vi "Write (Timestamp).vi"(9 "error in (no error)":errorcluster, 10 "Timestamp Value":timestamp, 11 "Config Element in":refnum<class "Config Element.lvclass">) -> (1 "error out":errorcluster, 3 "Config Element out":refnum<class "Config Element.lvclass">)   [LabVIEW 2020, in "CDM-Config.lvlib" / "Config Element.lvclass"]
uses:
  Config Element.lvclass
  CDM-Config.lvlib
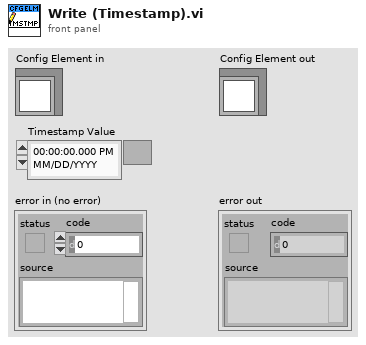
[diagram p1: front panel]
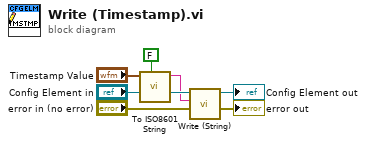
[diagram p0: block diagram]
diagram:
  n1 = call "To ISO8601 String.vi"("Now for Unset? (T)"=FALSE, "Time Stamp"="Timestamp Value") -> ("ISO 8601 UTC"=w2:string)  [unwired: 9 in]
  n2 = call "Write (String).vi"("error in (no error)"="error in (no error)", "String Value"=w2, "Config Element in"="Config Element in") -> ("error out"=→"error out":errorcluster, "Config Element out"=→"Config Element out":refnum<class "Config Element.lvclass">)  [unwired: 7 in]
